vi "RTS Send Custom Command.vi"(8 "Error In":errorcluster, 10 "Custom Commands":string[](array[string]), 11 "Read Door CMD in":string) -> (0 "Error Out":errorcluster, 3 "States":string)   [LabVIEW 2016]
uses:
  Type Definitions/RTS TCP Commands.ctl
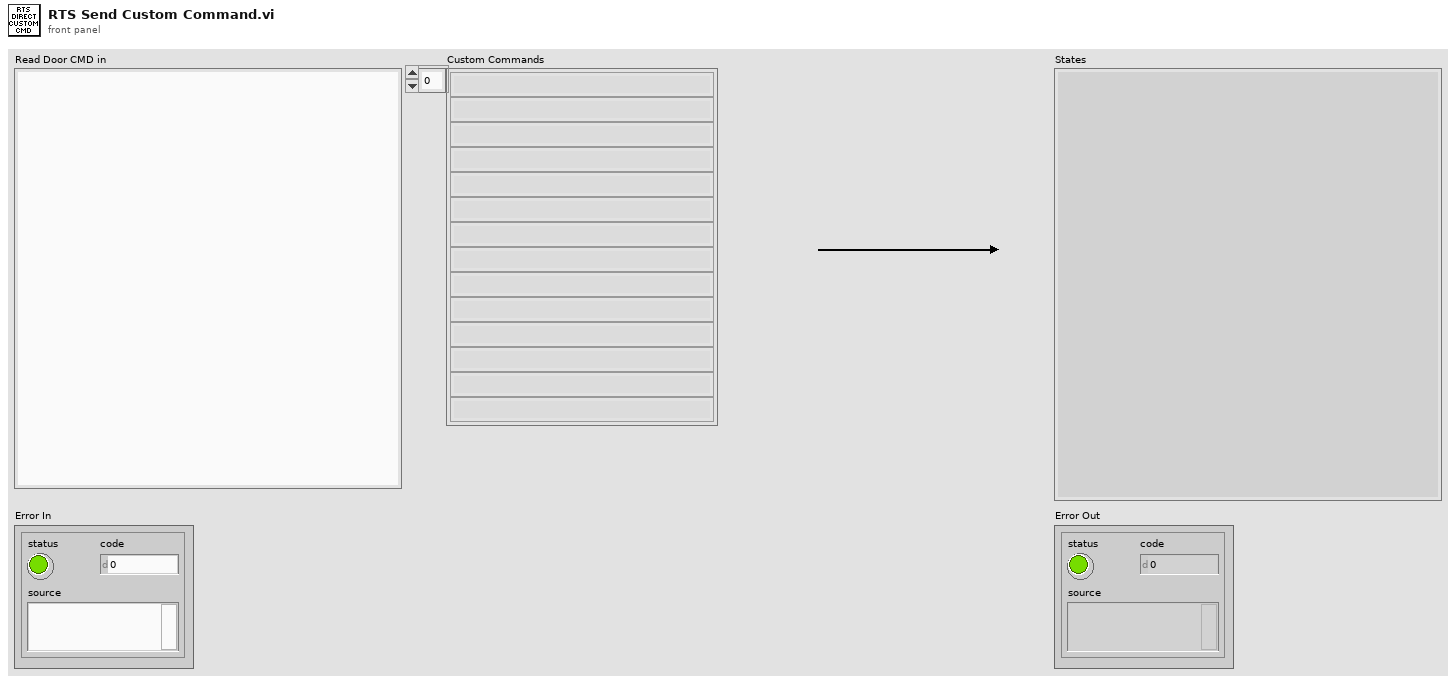
[diagram p1: front panel]
types:
  T1 = typedef "RTS TCP Commands.ctl" = string
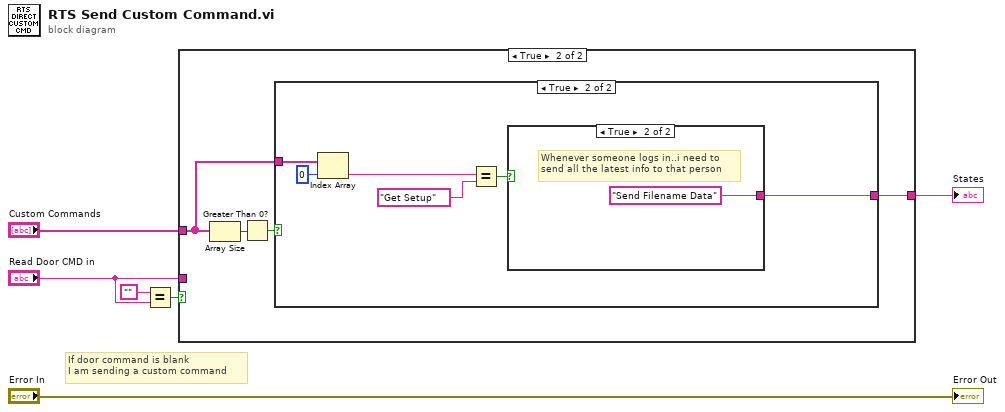
[diagram p0: block diagram]
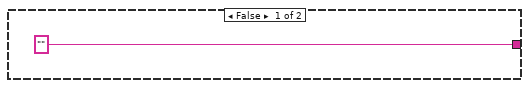
[diagram p3: hidden frame]
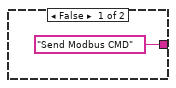
[diagram p4: hidden frame]
diagram:
  # "If door command is blank\nI am sending a custom command"
  n1 = Equal?(x="", y="Read Door CMD in") -> (x = y?=w5:bool)
  n2 = case shown="True" w5 {
    tunnel: "Custom Commands" -> [_ w8]
    tunnel: [w7 w9] -> w3
    tunnel: "Read Door CMD in" -> [w7 _]
    frame False {
    }
    frame True {
      n3 = Array Size(array=w8) -> (size(s)=w11:i32)
      n4 = Greater Than 0?(x=w11) -> (x > 0?=w10:bool)
      n5 = case shown="True" w10 {
        tunnel: ["" w18] -> w9
        tunnel: w8 -> [_ w17]
        frame False {
        }
        frame True {
          n6 = Index Array(array=w17, index=0) -> (element=w13:string)
          n7 = Equal?(x=w13, y=T1 "Get Setup" ("TCP Commands")) -> (x = y?=w15:bool)
          n8 = case shown="True" w15 {
            tunnel: ["Send Modbus CMD" "Send Filename Data"] -> w18
            frame False {
            }
            frame True {
              # "Whenever someone logs in..i need to \nsend all the latest info to that person"
            }
          }
        }
      }
    }
  }
  "States" <- w3
  "Error Out" <- "Error In"
